vi "Log Errors.vi"(7 "System":string="Source", 8 "error in":errorcluster, 11 "Time Stamp":timestamp) -> (0 "error out":errorcluster)   [LabVIEW 2013, in "Error Logger.lvclass"]
uses:
  Error Logger.lvclass
  Error Logger.lvclass/Error Logger.ctl
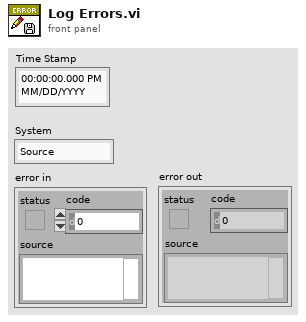
[diagram p1: front panel]
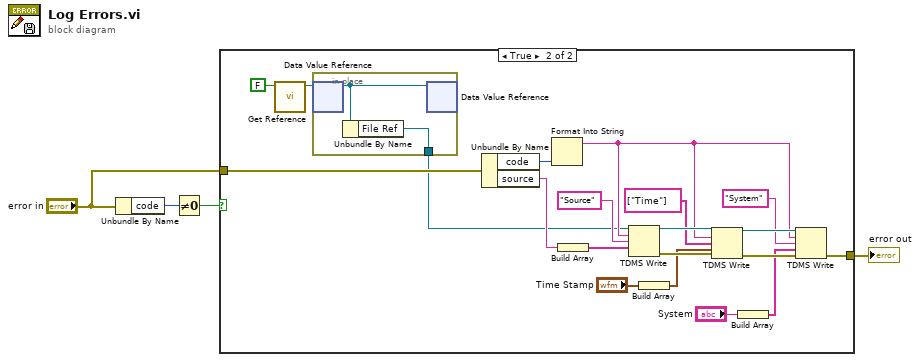
[diagram p0: block diagram]
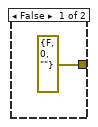
[diagram p2: hidden frame]
diagram:
  n1 = Unbundle By Name("error in") -> ("code"=w3:i32)
  n2 = Not Equal To 0?(x=w3) -> (x != 0?=w4:bool)
  n3 = case shown="True" w4 {
    tunnel: "error in" -> [_ w16]
    tunnel: [errorcluster {"status"=FALSE, "code"=0, "source"=""} ("error out") w6] -> w1
    frame False {
    }
    frame True {
      n4 = call "Get Reference.vi"("Init?"=FALSE) -> ("DVR"=w9:refnum<data-value>)  [unwired: 9 in, 1 out]
      n5 = in-place {
        in-place-border: [w27] -> w8
        n6 = in-place-dvr #1(w9) -> (w26:refnum<class "Error Logger.lvclass">)  [unwired: 1 out]
        n7 = Unbundle By Name(w26) -> ("File Ref"=w27:refnum<k34>)
        n8 = in-place-dvr #1(w26) -> ()  [unwired: 2 out]
      }
      n9 = Unbundle By Name(w16) -> ("code"=w25:i32, "source"=w24:string)
      n10 = Format Into String(w25) -> (resulting string=w13:string)  [unwired: 3 in, 1 out]
      n11 = Build Array(w24) -> (w23:string[])
      n12 = TDMS Write(0:w8, 5:w13, 7:"Source" ("channel name(s) in (Untitled)"), 9:w23) -> (4:w21:refnum<k34>, 15:w20:errorcluster)  [unwired: 2 in, 2 out]
      n13 = Build Array("Time Stamp") -> (w19:timestamp[])
      n14 = TDMS Write(0:w21, 5:w13, 7:string[] ["Time"] ("channel name(s) in (Untitled)"), 9:w19, 11:w20) -> (4:w15:refnum<k34>, 15:w14:errorcluster)  [unwired: 1 in, 2 out]
      n15 = Build Array("System") -> (w11:string[])
      n16 = TDMS Write(0:w15, 5:w13, 7:"System" ("channel name(s) in (Untitled)"), 9:w11, 11:w14) -> (15:w6:errorcluster)  [unwired: 1 in, 3 out]
    }
  }
  "error out" <- w1
